vi "Calibrate Path.vi"(8 "error in (no error)":errorcluster, 10 "Names":string[](array[string]), 11 "PathControl in":refnum<class "PathControl.lvclass">) -> (0 "error out":errorcluster, 2 "Canceled?":bool, 3 "PathControl out":refnum<class "PathControl.lvclass">)   [LabVIEW 2020, in "PathControl.lvclass"]
uses:
  PathControl.lvclass
  PathControl.lvclass/PathControl.ctl
  Instruments/Vector Network Analyzer/Controls/S parm format enum.ctl
  Instruments/Vector Network Analyzer/Vector Network Analyzer.lvclass
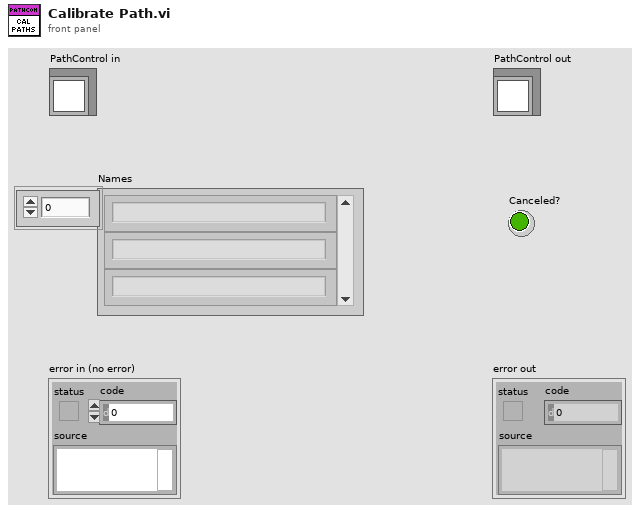
[diagram p1: front panel]
types:
  T1 = typedef "Vector Network Analyzer.lvclass/S parm format enum.ctl" = enum16{"Mag dB", "Mag", "Phase", "Smith", "Real", "Imag", "Group Delay", "SWR"}
  T2 = enum16{"S11", "S21", "S31", "S41", "S22", "S12", "S32", "S42", "S33", "S13", "S23", "S43", "S44", "S14", "S24", "S34"}
  T3 = cluster{"Name":string, "Path Frequency":dbl[], "Path Loss":dbl[]}
  T4 = cluster{"Name":string, "Path Frequency":dbl[], "Path Loss":dbl[]}[]
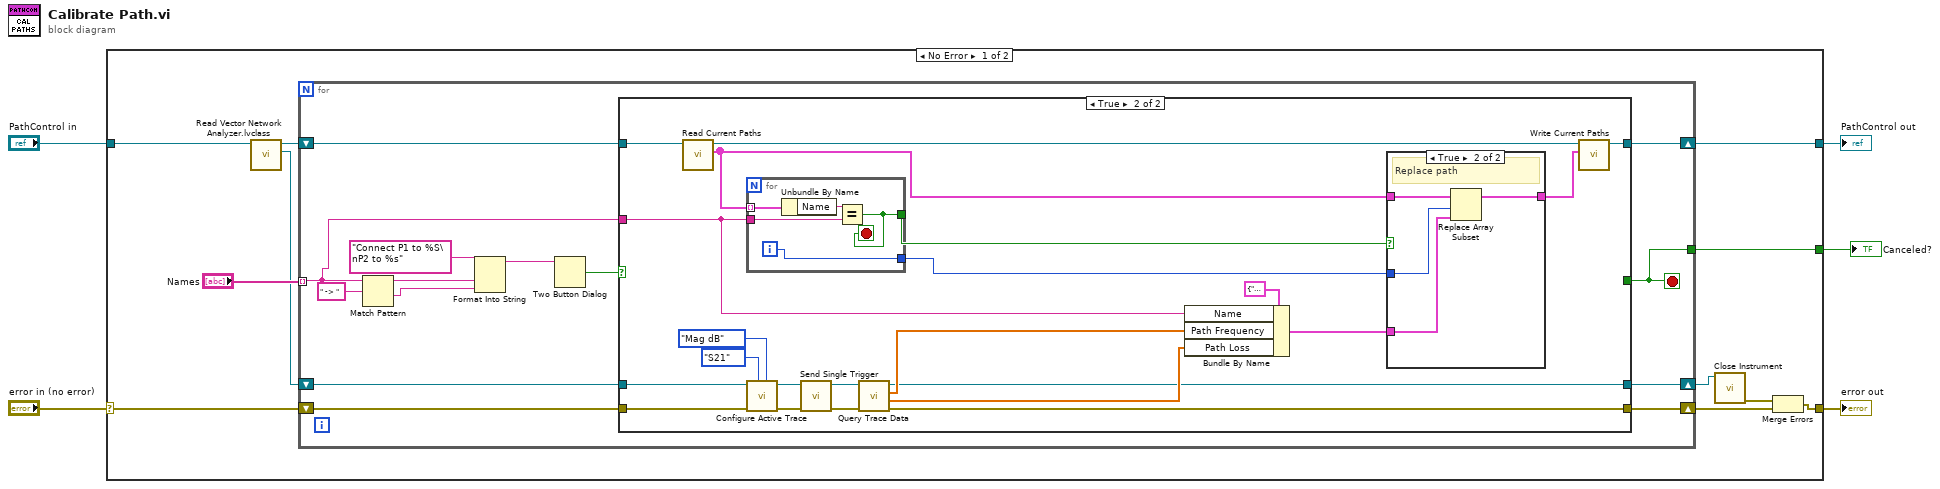
[diagram p0: block diagram]
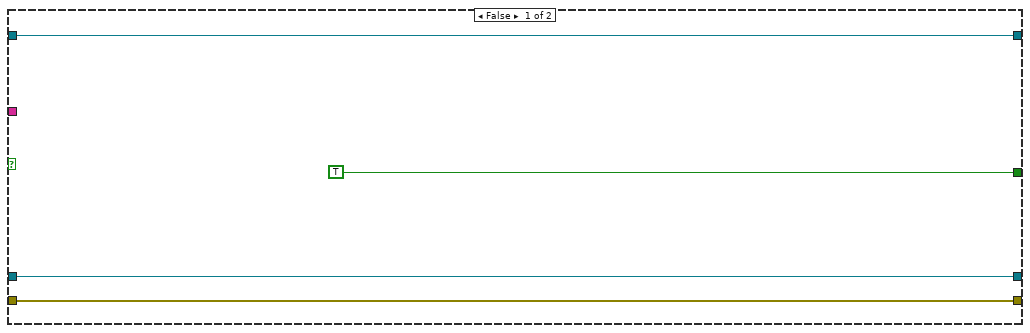
[diagram p2: hidden frame]
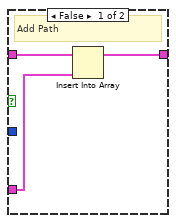
[diagram p3: hidden frame]
diagram:
  n1 = case shown="No Error" "error in (no error)" {
    selector: "error in (no error)" -> [w16 w70]
    tunnel: [w8 w70] -> w4
    tunnel: [w11 w69] -> w2
    tunnel: "PathControl in" -> [w14 w69]
    tunnel: [w10 _] -> w1
    frame No Error {
      n2 = call "Read Vector Network Analyzer.lvclass.vi"("PathControl in"=w14) -> ("Vector Network Analyzer.lvclass"=w13:refnum<class "Vector Network Analyzer.lvclass">, "PathControl out"=w12:refnum<class "PathControl.lvclass">)  [unwired: 9 in]
      n3 = for {
        shift-right: [w20] -> w9
        shift-left: w16 -> [w24]
        tunnel: "Names" -> [w23] mode=indexing
        shift-right: [w21] -> w11
        shift-left: w12 -> [w22]
        tunnel: [w19] -> w10
        shift-right: [w17] -> w6
        shift-left: w13 -> [w18]
        stop <- w19 stop-if-true
        n4 = Match Pattern(string=w23, regular expression=" -> ") -> (before substring=w28:string, after substring=w27:string)  [unwired: 1 in, 2 out]
        n5 = Format Into String(format string="Connect P1 to %S\nP2 to %s", w28, w27) -> (resulting string=w26:string)  [unwired: 2 in, 1 out]
        n6 = Two Button Dialog(message=w26) -> (T button?=w25:bool)  [unwired: 2 in]
        n7 = case shown="True" w25 {
          tunnel: w24 -> [w32 w44]
          tunnel: [TRUE _] -> w19
          tunnel: w18 -> [w31 w43]
          tunnel: w23 -> [_ w54]
          tunnel: w22 -> [w33 w56]
          tunnel: [w33 w49] -> w21
          tunnel: [w32 w36] -> w20
          tunnel: [w31 w35] -> w17
          frame False {
          }
          frame True {
            n8 = call "Read Current Paths.vi"("PathControl in"=w56) -> ("Current Paths"=w51:T4, "PathControl out"=w48:refnum<class "PathControl.lvclass">)  [unwired: 9 in]
            n9 = for {
              tunnel: w51 -> [w64] mode=indexing
              tunnel: w54 -> [w67]
              tunnel: [w66] -> w52
              tunnel: [w65] -> w53
              i -> [w66]
              stop <- w65 stop-if-true
              n10 = Unbundle By Name(w64) -> ("Name"=w68:string)
              n11 = Equal?(x=w68, y=w67) -> (x = y?=w65:bool)
            }
            n12 = call-dynamic "Configure Active Trace.vi"("Format"=S_parm_format_enum."Mag dB", "S parameter"=T2."S21", "error in (no error)"=w44, "Vector Network Analyzer in"=w43) -> ("error out"=w42:errorcluster, "Vector Network Analyzer out"=w41:refnum<class "Vector Network Analyzer.lvclass">)  [unwired: 6 in]
            n13 = call-dynamic "Send Single Trigger.vi"("error in (no error)"=w42, "Vector Network Analyzer in"=w41) -> ("error out"=w40:errorcluster, "Vector Network Analyzer out"=w39:refnum<class "Vector Network Analyzer.lvclass">)  [unwired: 8 in]
            n14 = call-dynamic "Query Trace Data.vi"("error in (no error)"=w40, "Vector Network Analyzer in"=w39) -> ("error out"=w36:errorcluster, "Data"=w37:dbl[], "Frequency"=w38:dbl[], "Vector Network Analyzer out"=w35:refnum<class "Vector Network Analyzer.lvclass">)  [unwired: 6 in]
            n15 = Bundle By Name(cluster=T3 {"Name"="", "Path Frequency"=[], "Path Loss"=[]} ("Path"), "Name"=w54, "Path Frequency"=w38, "Path Loss"=w37) -> (w50:T3)
            n16 = case shown="True" w53 {
              tunnel: w52 -> [_ w61]
              tunnel: w51 -> [w59 w63]
              tunnel: w50 -> [w58 w60]
              tunnel: [w57 w62] -> w47
              frame False {
                # "Add Path"
                n17 = Insert Into Array(array=w59, new element=w58) -> (w57:T4)  [unwired: 1 in]
              }
              frame True {
                # "Replace path"
                n18 = Replace Array Subset(array=w63, new element=w60, index=w61) -> (w62:T4)
              }
            }
            n19 = call "Write Current Paths.vi"("Current Paths"=w47, "PathControl in"=w48) -> ("PathControl out"=w49:refnum<class "PathControl.lvclass">)  [unwired: 9 in]
          }
        }
      }
      n20 = call-dynamic "Close Instrument.vi"("Instrument in"=w6) -> ("error out"=w7:errorcluster)  [unwired: 9 in, 1 out]
      n21 = Merge Errors(w7, w9) -> (w8:errorcluster)
    }
    frame Error {
    }
  }
  "error out" <- w4
  "PathControl out" <- w2
  "Canceled?" <- w1
